vi "Open.vi"(8 "error in (no error)":errorcluster, 11 "TCP Comm":T1) -> (0 "error out":errorcluster)   [LabVIEW 2020, in "TinyTCP.lvlib"]
doc: "Note: <b>Connection Loop.vi</b> must be running (either directly in parallel on a block diagram or launched with <b>Launch Connection Async.vi</b>) for a connection to actually open.\n\nStarts the connecting process. The connection process can be monitored with <b>Get State.vi</b> and <b>Get Connected.vi</b>"
uses:
  TinyTCP.lvlib
  Instance.ctl
  Ref Data.ctl
  State.ctl
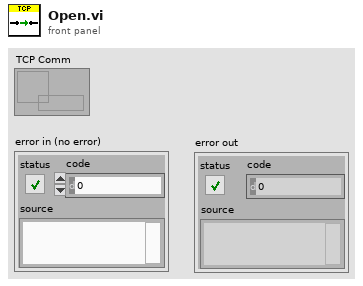
[diagram p1: front panel]
types:
  T1 = typedef "TinyTCP.lvlib/Instance.ctl" = refnum<data-value>
  T2 = typedef "TinyTCP.lvlib/State.ctl" = enum16{"Idle", "Starting", "Connecting", "Connected", "Disconnecting", "Stopped"}
  T3 = typedef "TinyTCP.lvlib/Ref Data.ctl" = cluster{"TCP":refnum<k5>, "State":T2, "Server":bool, "Host":string, "Port":u16, "Listener":refnum<k5>, "Start":bool, "Disconnect":bool, "TCP Valid":bool, "TLS Enabled":bool, "Immutable TLS":refnum<k36>, "Certificate DN":string}
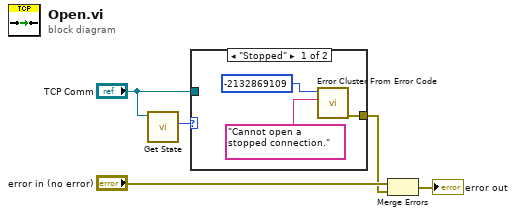
[diagram p0: block diagram]
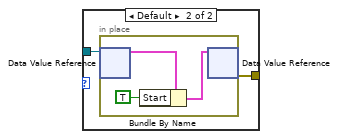
[diagram p2: hidden frame]
diagram:
  n1 = call "Get State.vi"("TCP Comm In"="TCP Comm") -> ("State"=w2:T2)  [unwired: 9 in, 1 out]
  n2 = case shown="\"Stopped\"" w2 {
    tunnel: [w8 w10] -> w4
    tunnel: "TCP Comm" -> [_ w9]
    frame "Stopped" {
      n3 = call <vilib>:"Error Cluster From Error Code.vi"("error message (\"\")"="Cannot open a stopped connection." ("error message (\"\")"), "error code (0)"=-2132869109) -> ("error out"=w8:errorcluster)  [unwired: 7 in]
    }
    frame Default {
      n4 = in-place {
        n5 = in-place-dvr #1(w9) -> (w13:T3)  [unwired: 1 out]
        n6 = Bundle By Name(cluster=w13, "Start"=TRUE) -> (w12:T3)
        n7 = in-place-dvr #1(w12) -> (w10:errorcluster)  [unwired: 1 out]
      }
    }
  }
  n8 = Merge Errors("error in (no error)", w4) -> (→"error out":errorcluster)
